vi "PNDT - waveform decoder.vi"(8 "header (1A)":u8=26 format="%.0x", 10 "[U8]":u8[](array[numeric]) format="%02x", 11 "DOF":T2=enum."8-bit Mode" caption="dof") -> (0 "scan data":u16[](array[numeric]) format="%04x", 1 "retain data":T1=enum."Ascan", 2 "#peaks":i32, 3 "XY data":cluster{u16[], u16[]})   [LabVIEW 2026, in "MicroPulse_Driver.lvlib"]
uses:
  MicroPulse_Driver.lvlib
  Public/Data/Datatypes/MP - data output format.ctl
  Public/Data/Datatypes/MP - retain scan.ctl
panel:
  # "[array]"
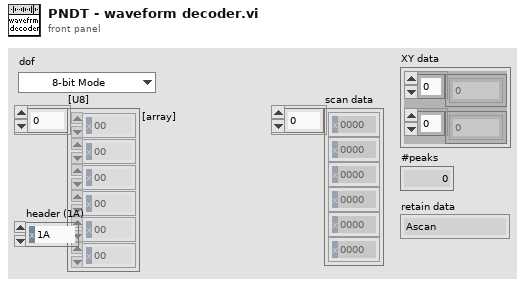
[diagram p1: front panel]
types:
  T1 = typedef "MicroPulse_Driver.lvlib/MP - retain scan.ctl" = enum16{"None", "Ascan", "Peaks"}
  T2 = typedef "MicroPulse_Driver.lvlib/MP - data output format.ctl" = enum16{"", "8-bit Mode", "10-bit Mode", "12-bit Mode", "16-bit Mode", "8-bit Log Mode", "12-bit Packed Mode"}
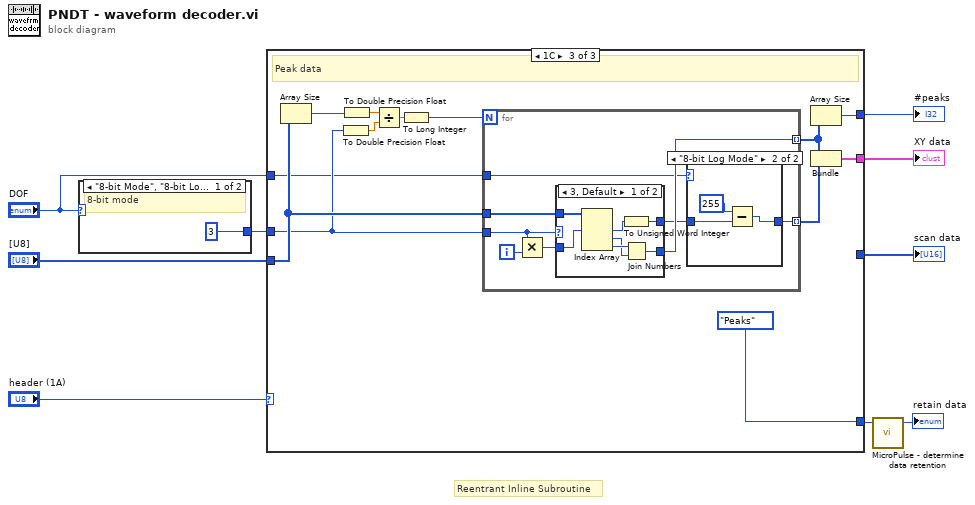
[diagram p0: block diagram]
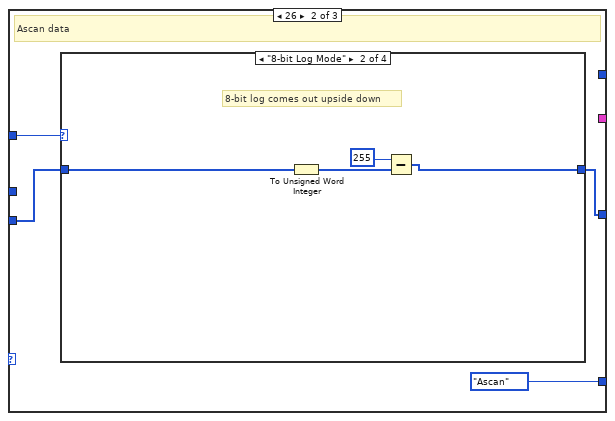
[diagram p3: hidden frame]
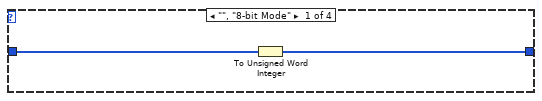
[diagram p4: hidden frame]
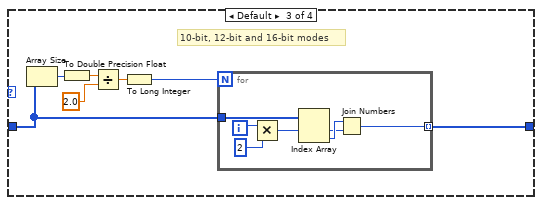
[diagram p5: hidden frame]
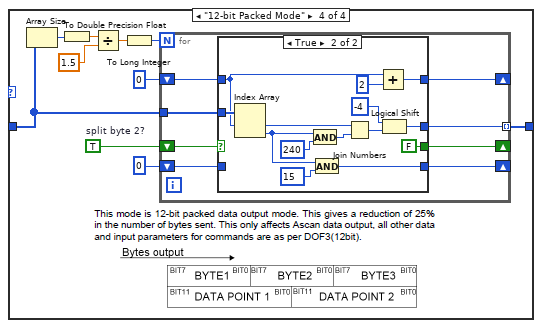
[diagram p6: hidden frame]
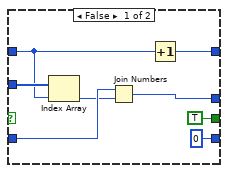
[diagram p7: hidden frame]
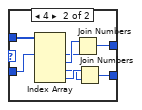
[diagram p9: hidden frame]
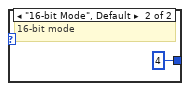
[diagram p10: hidden frame]
diagram:
  # "Reentrant Inline Subroutine"
  n1 = case shown="\"8-bit Mode\", \"8-bit Log Mode\"" "DOF" {
    tunnel: [3 ("x") 4 ("x")] -> w6
    frame "8-bit Mode", "8-bit Log Mode" {
      # "8-bit mode"
    }
    frame "16-bit Mode", Default {
      # "16-bit mode"
    }
  }
  n2 = case shown="1C" "header (1A)" {
    tunnel: [_ w13 _] -> w5
    tunnel: "[U8]" -> [_ w15 w84]
    tunnel: [_ MP_-_retain_scan."Ascan" ("scan type") MP_-_retain_scan."Peaks" ("scan type")] -> w2
    tunnel: "DOF" -> [_ w14 w76]
    tunnel: w6 -> [_ _ w83]
    tunnel: [_ _ w82] -> w4
    tunnel: [_ _ w80] -> w3
    frame Default {
    }
    frame 26 {
      # "Ascan data"
      n3 = case shown="\"8-bit Log Mode\"" w14 {
        tunnel: [w17 w19 w22 w39] -> w13
        tunnel: w15 -> [w16 w20 w27 w44]
        frame "", "8-bit Mode" {
          n4 = To Unsigned Word Integer(number=w16) -> (unsigned 16bit integer=w17:u16[])
        }
        frame "8-bit Log Mode" {
          # "8-bit log comes out upside down"
          n5 = To Unsigned Word Integer(number=w20) -> (unsigned 16bit integer=w21:u16[])
          n6 = Subtract(x=u16 255, y=w21) -> (x-y=w19:u16[])
        }
        frame Default {
          # "10-bit, 12-bit and 16-bit modes"
          n7 = Array Size(array=w27) -> (size(s)=w23:i32)
          n8 = To Double Precision Float(number=w23) -> (double precision float=w26:dbl)
          n9 = Divide(x=w26, y=2.0) -> (x/y=w24:dbl)
          n10 = To Long Integer(number=w24) -> (32bit integer=w28:i32)
          n11 = for {
            N: w28 -> [_]
            tunnel: w27 -> [w35]
            tunnel: [w29] -> w22 mode=indexing
            i -> [w31]
            n12 = Multiply(x=w31, y=2) -> (x*y=w30:i32)
            n13 = Index Array(array=w35, index #1=w30) -> (element #1=w33:u8, element #2=w34:u8)  [unwired: 1 in]
            n14 = Join Numbers(hi=w34, lo=w33) -> ((hi.lo)=w29:u16)
          }
        }
        frame "12-bit Packed Mode" {
          w36 = TRUE  # split byte 2?
          n15 = Array Size(array=w44) -> (size(s)=w40:i32)
          n16 = To Double Precision Float(number=w40) -> (double precision float=w43:dbl)
          n17 = Divide(x=w43, y=1.5) -> (x/y=w41:dbl)
          n18 = To Long Integer(number=w41) -> (32bit integer=w45:i32)
          n19 = for {
            N: w45 -> [_]
            tunnel: w44 -> [w53]
            tunnel: [w52] -> w39 mode=indexing
            shift-right: [w50] -> _
            shift-left: u8 0 ("U8") -> [w51]
            shift-right: [w48] -> _
            shift-left: 0 -> [w49]
            shift-right: [w46] -> _
            shift-left: w36 -> [w47]
            n20 = case shown="True" w47 {
              tunnel: w53 -> [w61 w75]
              tunnel: [w56 w68] -> w52
              tunnel: w51 -> [w58 _]
              tunnel: [u8 0 w63] -> w50
              tunnel: w49 -> [w60 w66]
              tunnel: [w59 w64] -> w48
              tunnel: [TRUE FALSE] -> w46
              frame False {
                n21 = Index Array(array=w61, index=w60) -> (element=w57:u8)
                n22 = Join Numbers(hi=w58, lo=w57) -> ((hi.lo)=w56:u16)
                n23 = Increment(x=w60) -> (x+1=w59:i32)
              }
              frame True {
                n24 = Index Array(array=w75, index #1=w66) -> (element #1=w70:u8, element #2=w74:u8)  [unwired: 1 in]
                n25 = And(x=w74, y=u8 240) -> (x .and. y?=w71:u8)
                n26 = And(x=w74, y=u8 15) -> (x .and. y?=w63:u8)
                n27 = Join Numbers(hi=w70, lo=w71) -> ((hi.lo)=w69:u16)
                n28 = Add(x=w66, y=2) -> (x+y=w64:i32)
                n29 = Logical Shift(y=i16 -4, x=w69) -> (x << y=w68:u16)
              }
            }
          }
        }
      }
    }
    frame 28 {
      # "Peak data"
      n30 = Array Size(array=w84) -> (size(s)=w87:i32)
      n31 = To Double Precision Float(number=w83) -> (double precision float=w86:dbl)
      n32 = To Double Precision Float(number=w87) -> (double precision float=w88:dbl)
      n33 = Divide(x=w88, y=w86) -> (x/y=w85:dbl)
      n34 = To Long Integer(number=w85) -> (32bit integer=w81:i32)
      n35 = for {
        N: w81 -> [_]
        tunnel: w84 -> [w96]
        tunnel: w83 -> [w95]
        tunnel: [w93] -> w78 mode=indexing
        tunnel: [w90] -> w77 mode=indexing
        tunnel: w76 -> [w89]
        i -> [w91]
        n36 = Multiply(x=w95, y=w91) -> (x*y=w94:i32)
        n37 = case shown="3, Default" w95 {
          tunnel: w96 -> [w107 w115]
          tunnel: [w102 w113] -> w92
          tunnel: [w103 w114] -> w93
          tunnel: w94 -> [w101 w108]
          frame 3, Default {
            n38 = Index Array(array=w107, index #1=w101) -> (element #1=w106:u8, element #2=w104:u8, element #3=w105:u8)  [unwired: 2 in]
            n39 = To Unsigned Word Integer(number=w106) -> (unsigned 16bit integer=w102:u16)
            n40 = Join Numbers(hi=w105, lo=w104) -> ((hi.lo)=w103:u16)
          }
          frame 4 {
            n41 = Index Array(array=w115, index #1=w108) -> (element #1=w111:u8, element #2=w112:u8, element #3=w109:u8, element #4=w110:u8)  [unwired: 3 in]
            n42 = Join Numbers(hi=w112, lo=w111) -> ((hi.lo)=w113:u16)
            n43 = Join Numbers(hi=w110, lo=w109) -> ((hi.lo)=w114:u16)
          }
        }
        n44 = case shown="\"8-bit Log Mode\"" w89 {
          tunnel: w92 -> [w97 w100]
          tunnel: [w97 w99] -> w90
          frame "", Default {
          }
          frame "8-bit Log Mode" {
            n45 = Subtract(x=u16 255 ("y"), y=w100) -> (x-y=w99:u16)
          }
        }
      }
      n46 = Array Size(array=w78) -> (size(s)=w82:i32)
      n47 = Bundle(w78, w77) -> (w80:cluster{u16[], u16[]})  [unwired: 1 in]
    }
  }
  "scan data" <- w5
  "#peaks" <- w4
  "XY data" <- w3
  n48 = call "MicroPulse - determine data retention.vi"("retain scan"=w2) -> ("retain scan"=→"retain data":T1)  [unwired: 4 in]
